vi "templogger_dev.vi"(4 "Seconds":dbl=360.0) -> (0 "Temperature":dbl, 2 "Time":timestamp)   [LabVIEW 2017]
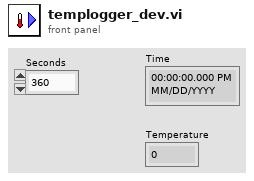
[diagram p1: front panel]
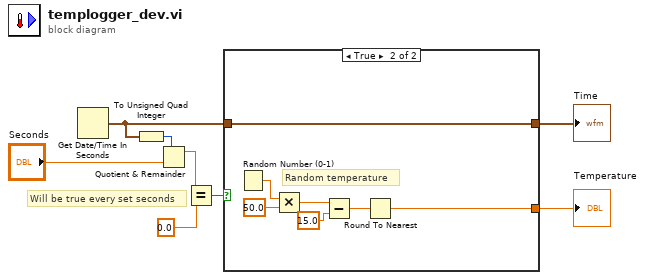
[diagram p0: block diagram]
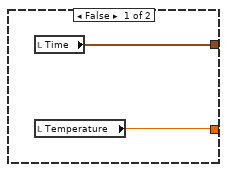
[diagram p2: hidden frame]
diagram:
  # "Will be true every set seconds"
  n1 = Get Date/Time In Seconds() -> (seconds since 1Jan1904=w4:timestamp)
  n2 = To Unsigned Quad Integer(1:w4) -> (0:w5:u64)
  n3 = Quotient & Remainder(x=w5, y="Seconds") -> (x-y*floor(x/y)=w6:dbl)  [unwired: 1 out]
  n4 = Equal?(x=w6, y=0.0) -> (x = y?=w8:bool)
  n5 = case shown="True" w8 {
    tunnel: w4 -> [_ w11]
    tunnel: [w10 w11] -> w1
    tunnel: [w9 w12] -> w2
    frame False {
      n6 = local read "Time"() -> (w10:timestamp)
      n7 = local read "Temperature"() -> (w9:dbl)
    }
    frame True {
      # "Random temperature"
      n8 = Random Number (0-1)() -> (number: 0 to 1=w16:dbl)
      n9 = Multiply(x=w16, y=50.0) -> (x*y=w17:dbl)
      n10 = Subtract(x=w17, y=15.0) -> (x-y=w13:dbl)
      n11 = Round To Nearest(number=w13) -> (nearest integer value=w12:dbl)
    }
  }
  "Temperature" <- w2
  "Time" <- w1
